vi "Convert 2D array from excel to cluster.vi"(11 "2D excel array":string[][](array[string])) -> (3 "Command Library as Array of Clusters":T1[](array[typedef]))   [LabVIEW 2020]
uses:
  Command Library Data.ctl
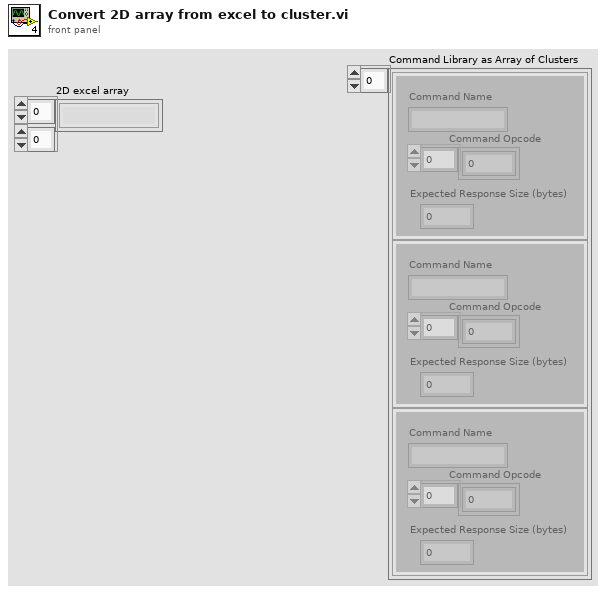
[diagram p1: front panel]
types:
  T1 = typedef "Command Library Data.ctl" = cluster{"Command Name":string, "Command Opcode":u8[], "Expected Response Size (bytes)":u16}
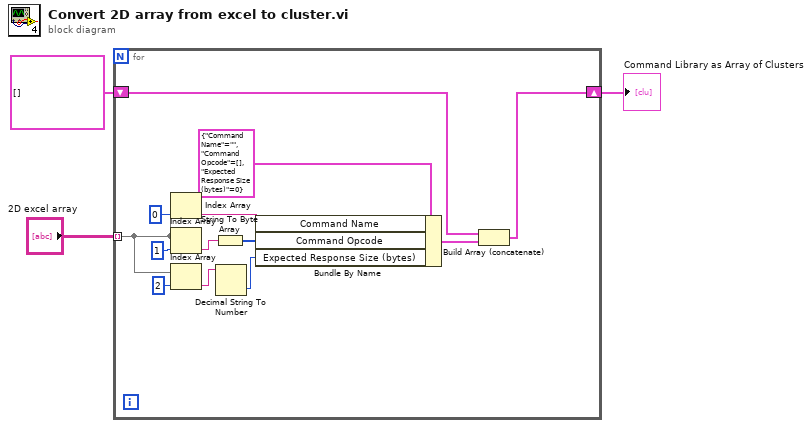
[diagram p0: block diagram]
diagram:
  n1 = for {
    tunnel: "2D excel array" -> [w13] mode=indexing
    shift-right: [w4] -> w1
    shift-left: T1[] [] -> [w5]
    n2 = Index Array(array=w13, index=0) -> (element=w12:string)
    n3 = Index Array(array=w13, index=1) -> (element=w10:string)
    n4 = Index Array(array=w13, index=2) -> (element=w8:string)
    n5 = String To Byte Array(string=w10) -> (unsigned byte array=w9:u8[])
    n6 = Decimal String To Number(string=w8) -> (number=w7:i32)  [unwired: 2 in, 1 out]
    n7 = Bundle By Name(cluster=T1 {"Command Name"="", "Command Opcode"=[], "Expected Response Size (bytes)"=0} ("Command Library Data"), "Command Name"=w12, "Command Opcode"=w9, "Expected Response Size (bytes)"=w7) -> (w6:T1)
    n8 = Build Array (concatenate)(w5, w6) -> (w4:T1[])
  }
  "Command Library as Array of Clusters" <- w1
